vi "Excel Write Text.vi"(6 "Text":string, 8 "error in":errorcluster caption="에러 입력(에러 없음)", 9 "Address in":cluster{"Row":i32, "Column":i32}, 11 "Excel._Worksheet in":refnum<k7>) -> (0 "error out":errorcluster caption="에러 출력", 1 "Below Cell":cluster{"Row":i32, "Column":i32}, 3 "Excel._Worksheet out":refnum<k7>)   [LabVIEW 2020]
panel:
  in  "Array":string[](array[string])=["A", "B", "C", "D", "E", "F", "G", "H", "I", "J", "K", "L", "M", "N", "O", "P", "Q", "R", "S", "T", "U", "V", "W", "X", "Y", "Z"]
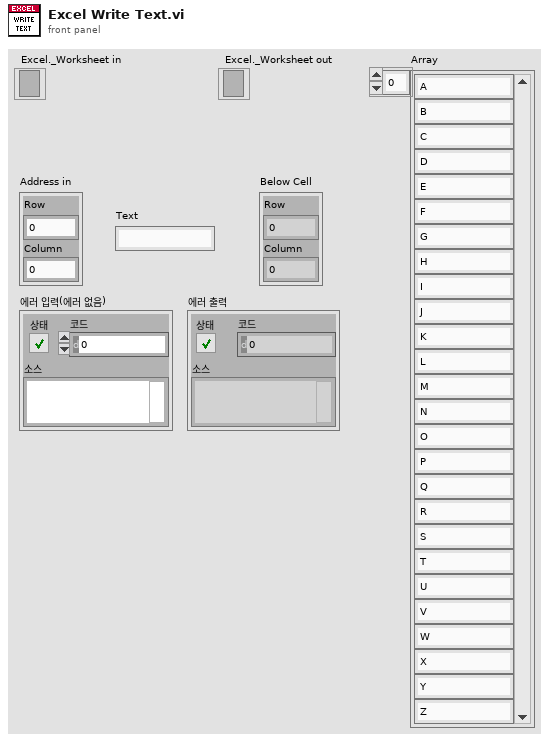
[diagram p1: front panel]
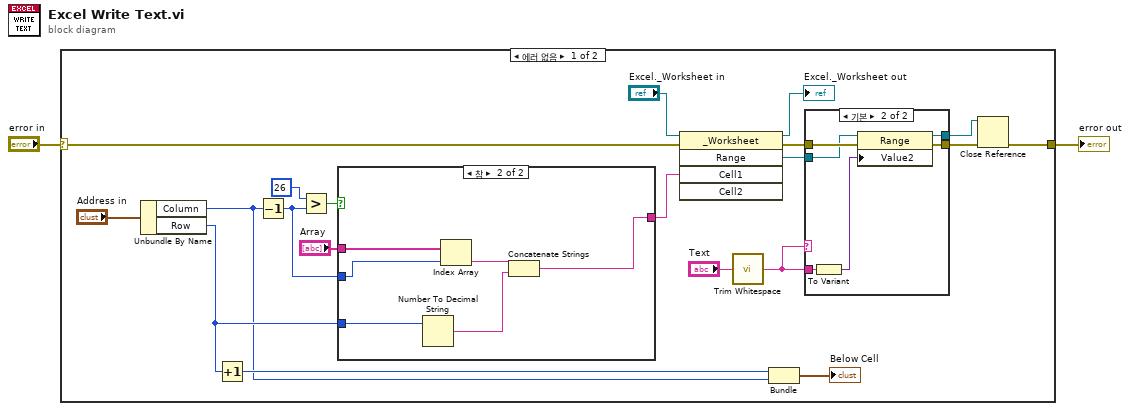
[diagram p0: block diagram]
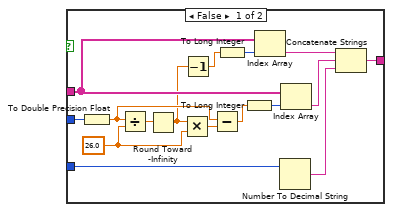
[diagram p3: hidden frame]
diagram:
  n1 = case shown="에러 없음" "error in" {
    selector: "error in" -> [w17 w53]
    tunnel: [w7 w53] -> w2
    frame No Error {
      n2 = Unbundle By Name("Address in") -> ("Column"=w3:i32, "Row"=w6:i32)
      n3 = Increment(x=w6) -> (x+1=w5:i32)
      n4 = Decrement(x=w3) -> (x-1=w4:i32)
      n5 = Greater?(x=26 ("y"), y=w4) -> (0:w15:bool)
      n6 = case shown="참" w15 {
        tunnel: "Array" -> [w42 w52]
        tunnel: w4 -> [w45 w51]
        tunnel: w6 -> [w39 w50]
        tunnel: [w37 w47] -> w12
        frame False {
          w31 = 26.0 ("y")
          n7 = To Double Precision Float(number=w45) -> (double precision float=w33:dbl)
          n8 = Divide(x=w33, y=w31) -> (x/y=w46:dbl)
          n9 = Round Toward -Infinity(1:w46) -> (0:w32:dbl)
          n10 = Multiply(x=w32, y=w31) -> (x*y=w44:dbl)
          n11 = Decrement(x=w32) -> (x-1=w36:dbl)
          n12 = Subtract(x=w33, y=w44) -> (x-y=w43:dbl)
          n13 = To Long Integer(number=w36) -> (32bit integer=w35:i32)
          n14 = To Long Integer(number=w43) -> (32bit integer=w34:i32)
          n15 = Index Array(array=w42, index=w35) -> (element=w41:string)
          n16 = Number To Decimal String(number=w39) -> (decimal integer string=w38:string)  [unwired: 1 in]
          n17 = Index Array(array=w42, index=w34) -> (element=w40:string)
          n18 = Concatenate Strings(w41, w40, w38) -> (w37:string)
        }
        frame True {
          n19 = Number To Decimal String(number=w50) -> (decimal integer string=w48:string)  [unwired: 1 in]
          n20 = Index Array(array=w52, index=w51) -> (element=w49:string)
          n21 = Concatenate Strings(w49, w48) -> (w47:string)
        }
      }
      n22 = invoke class="_Worksheet" method="Range"(reference="Excel._Worksheet in", error in=w17, "Cell1"=w12) -> (reference out=→"Excel._Worksheet out":refnum<k7>, error out=w20:errorcluster, "Range"=w19:refnum<k7>)  [unwired: 2 in, 2 out]
      n23 = call <vilib>:"Trim Whitespace.vi"("string"="Text") -> ("trimmed string"=w11:string)  [unwired: 1 in]
      n24 = Bundle(w5, "Column"=w3) -> (→"Below Cell":cluster{i32, "Column":i32})  [unwired: 1 in]
      n25 = case shown="기본" w11 {
        tunnel: w20 -> [w23 w30]
        tunnel: w19 -> [w24 w29]
        tunnel: [w24 w27] -> w9
        tunnel: [w23 w26] -> w8
        tunnel: w11 -> [_ w25]
        frame "" {
        }
        frame Default {
          n26 = To Variant(anything=w25) -> (Variant=w28:variant)
          n27 = property class="Range"(reference=w29, error in=w30, "Value2"=w28) -> (reference out=w27:refnum<k7>, error out=w26:errorcluster)
        }
      }
      n28 = Close Reference(reference=w9, error in (no error)=w8) -> (error out=w7:errorcluster)
    }
    frame Error {
    }
  }
  "error out" <- w2
